vi "DELETE Stop Event.vi"   [LabVIEW 2013]
uses:
  Functional Globals/Action.ctl
  Event Selector.ctl
types:
  T1 = typedef "Event Selector.ctl" = enum16{"Stop", "Reload Config"}
  T2 = typedef "Action.ctl" = enum16{"GET", "PUT", "DELETE"}
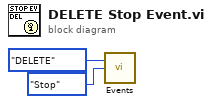
[diagram p0: block diagram]
diagram:
  n1 = call "Events.vi"("Event Type"=Event_Selector."Stop", "Action"=Action."DELETE") -> ()  [unwired: 1 in, 1 out]
